vi "Read Execution time.vi"(11 "Test Case Result In":refnum<class "Test Case Result.lvclass">) -> (2 "Execution time":dbl, 3 "Test Case Result Out":refnum<class "Test Case Result.lvclass">)   [LabVIEW 2020, in "Test Case Result.lvclass"]
uses:
  Test Case Result.lvclass
  Test Case Result.lvclass/Test Case Result.ctl
  Method Result/Method Result.lvclass/Method Result.ctl
  Method Result/Method Result.lvclass
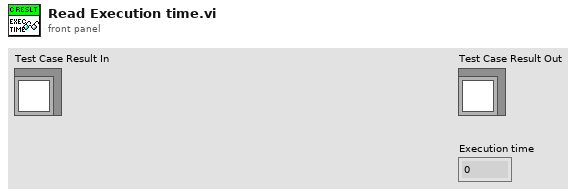
[diagram p1: front panel]
types:
  T1 = map{string, refnum<class "Method Result.lvclass">}
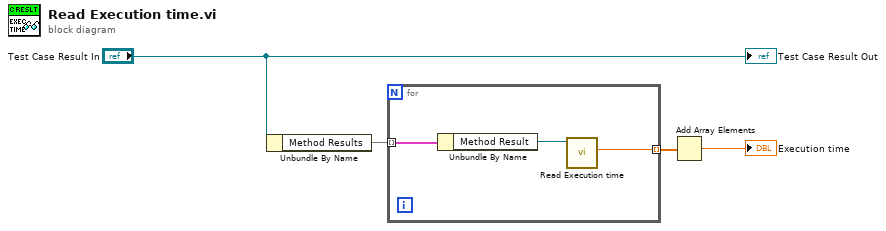
[diagram p0: block diagram]
diagram:
  n1 = Unbundle By Name("Test Case Result In") -> ("Method Results"=w3:T1)
  n2 = for {
    tunnel: w3 -> [w5] mode=indexing
    tunnel: [w7] -> w2 mode=indexing
    n3 = Unbundle By Name(w5) -> ("Method Result"=w6:refnum<class "Method Result.lvclass">)
    n4 = call "Read Execution time.vi"("Method Result In"=w6) -> ("Execution time"=w7:dbl)  [unwired: 8 in, 2 out]
  }
  n5 = Add Array Elements(numeric array=w2) -> (sum=→"Execution time":dbl)
  "Test Case Result Out" <- "Test Case Result In"
